vi "ctx get next access point record list.vi"(11 "context":u32) -> (2 "function return":i32, 3 "context out":u32)   [LabVIEW 2019, in "apdm.lvlib"]
doc: "APDM_EXPORT int apdm_ctx_get_next_access_point_record_list(apdm_ctx_t context);"
uses:
  apdm.lvlib
  Lee Lab/CP FES Walking 2018/Code/Working/LabVIEW/apdm.dll
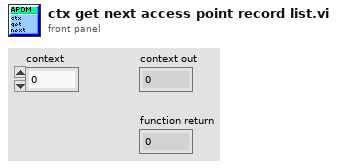
[diagram p1: front panel]
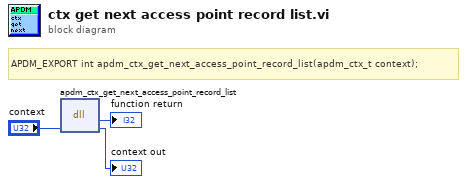
[diagram p0: block diagram]
diagram:
  # "APDM_EXPORT int apdm_ctx_get_next_access_point_record_list(apdm_ctx_t context);"
  n1 = dll-call lib="C:/Users/jfalesi/Dropbox/Lee Lab/CP FES Walking 2018/Code/Working/LabVIEW/apdm.*" fn="apdm_ctx_get_next_access_point_record_list"("context"="context") -> (→"function return":i32, "context"=→"context out":u32)  [unwired: 3 in, 2 out]
